vi "LV86_Morph_Open.vi"(2 "Connectivity":enum16{"4", "6", "8"}(ring), 3 "Image in":T1 {"Dialogs" format="%.0b"}) -> (1 "Image out":T1 {"Dialogs" format="%.0b"})   [LabVIEW 2024]
doc: "This VI removes bright spots isolated in dark regions and smooths boundaries."
uses:
  <userlib>/ImageProcessing/QTLIB_2595_LV86/QT_Image.ctl
panel:
  out "Open morph":picture caption="new picture"
  out "Initial Image":picture caption="new picture"
  # "This VI removes bright spots isolated in dark regions \nand smooths boundaries."
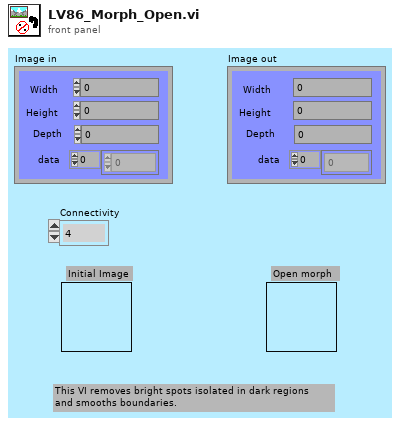
[diagram p1: front panel]
types:
  T1 = typedef "QT_Image.ctl" = cluster{"Width":i32, "Height":i32, "Depth":i32, "data":u8[], "Compressed data":u8[], "Color table":u32[], "Duration":i32, "Options":i32, "Timestamp":i32, "ID":i32, "Reserved":i32, "Dialogs":u32}
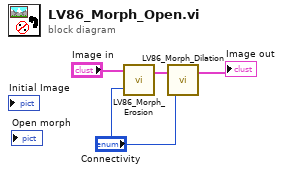
[diagram p0: block diagram]
diagram:
  n1 = call <userlib>:"LV86_Morph_Erosion.vi"("Connectivity"="Connectivity", "Image in"="Image in") -> ("Image out"=w3:T1)  [unwired: 1 out]
  n2 = call <userlib>:"LV86_Morph_Dilation.vi"("Connectivity"="Connectivity", "Image in"=w3) -> ("Image out"=→"Image out":T1)  [unwired: 1 out]
